vi "Sniffer.vi"() -> ()   [LabVIEW 2017]
uses:
  <vilib>/Instr/_visa.llb/VISA Open Access Mode.ctl
  <vilib>/Instr/_visa.llb/VISA Configure Serial Port (Instr).vi
panel:
  in  "Start":bool caption="Play Button"
  in  "Refresh Button":bool
  out "String":string
  in  "Stop Button":bool
  in  "flow control (0:none)":u16(ring) items=["None", "XON/XOFF", "RTS/CTS", "XON/XOFF & RTS/CTS", "DTR/DSR", "XON/XOFF & DTR/DSR"]
  in  "stop bits (10: 1 bit)":u16=10
  in  "parity (0:none)":u16(ring) items=["None", "Odd", "Even", "Mark", "Space"]
  in  "data bits (8)":u16=8 min=5 max=8 step=1
  in  "baud rate (9600)":u32=460800
  in  "Enable Termination\nChar (T)":bool
  in  "termination char\n(0xA = '\\n' = LF)":u8=10 format="%.0x"
  in  "timeout (10sec)":u32=100
  in  "VISA resource name":refnum<visa-resource-name>="COM3"
  # "V 0.1c"
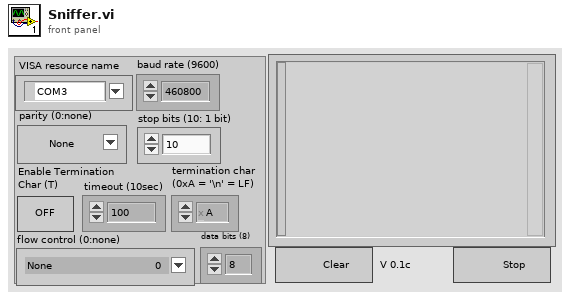
[diagram p1: front panel]
types:
  T1 = typedef "VISA Open Access Mode.ctl" = u32
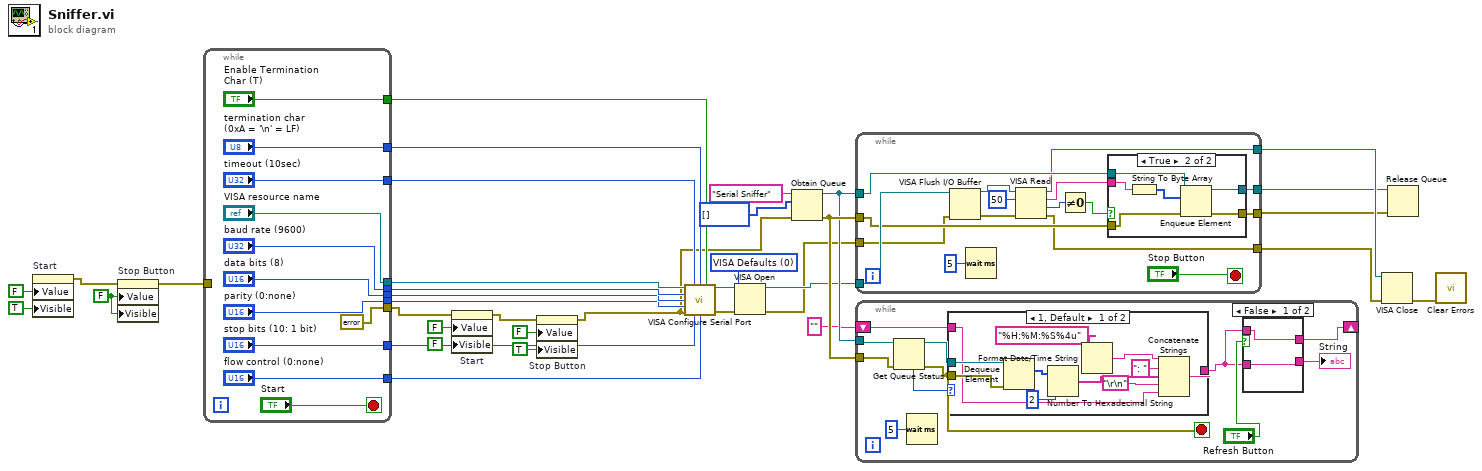
[diagram p0: block diagram]
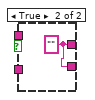
[diagram p2: hidden frame]
diagram:
  w12 = FALSE ("Stop Button")
  w25 = T1 0 items=["VISA Defaults"=0, "Exclusive Lock"=1, "Load Configured Settings"=4] ("Access Mode")
  n1 = property on="Start" class="Bool (strict)"("Value"=FALSE ("Start"), "Visible"=TRUE) -> (error out=w8:errorcluster)  [unwired: 2 in, 1 out]
  n2 = property on="Stop Button" class="Bool (strict)"(error in=w8, "Value"=w12, "Visible"=w12) -> (error out=w11:errorcluster)  [unwired: 1 in, 1 out]
  n3 = while {
    tunnel: ["VISA resource name"] -> w36
    tunnel: ["timeout (10sec)"] -> w35
    tunnel: ["termination char\n(0xA = '\\n' = LF)"] -> w34
    tunnel: ["baud rate (9600)"] -> w33
    tunnel: ["data bits (8)"] -> w32
    tunnel: ["parity (0:none)"] -> w31
    tunnel: ["stop bits (10: 1 bit)"] -> w30
    tunnel: ["flow control (0:none)"] -> w29
    tunnel: ["Enable Termination\nChar (T)"] -> w28
    tunnel: [errorcluster {"status"=FALSE, "code"=0, "source"=""} ("error in (no error)")] -> w3
    tunnel: w11 -> [_]
    stop <- "Start" stop-if-true
  }
  n4 = property on="Start" class="Bool (strict)"(error in=w3, "Value"=FALSE ("Start"), "Visible"=FALSE) -> (error out=w7:errorcluster)  [unwired: 1 in, 1 out]
  n5 = property on="Stop Button" class="Bool (strict)"(error in=w7, "Value"=FALSE ("Stop Button"), "Visible"=TRUE) -> (error out=w2:errorcluster)  [unwired: 1 in, 1 out]
  n6 = call-poly "VISA Configure Serial Port"("VISA resource name"=w36, "timeout (10sec)"=w35, "termination char\n(0xA = '\\n' = LF)"=w34, "Enable Termination\nChar (T)"=w28, "baud rate (9600)"=w33, "data bits (8)"=w32, "parity (0:none)"=w31, "error in (no error)"=w2, "stop bits (10: 1 bit)"=w30, "flow control (0:none)"=w29) -> ("VISA resource name out"=w27:refnum<visa-resource-name>, "error out"=w26:errorcluster)  [unwired: 4 in]
  n7 = VISA Open(access mode=w25, error in (no error)=w26, VISA resource name=w27) -> (VISA resource name=w21:refnum<visa-resource-name>, error out=w20:errorcluster)  [unwired: 2 in]
  n8 = Obtain Queue(name (unnamed)="Serial Sniffer", element data type=u8[] [], error in (no error)=w2) -> (queue out=w22:refnum<queue>, error out=w23:errorcluster)  [unwired: 2 in, 1 out]
  n9 = while {
    tunnel: w22 -> [w56]
    tunnel: w23 -> [w55]
    tunnel: w21 -> [w61]
    tunnel: [w54] -> w17
    tunnel: w20 -> [w53]
    tunnel: [w51] -> w19
    tunnel: [w50] -> w18
    tunnel: [w49] -> w16
    stop <- "Stop Button" stop-if-true
    n10 = VISA Flush I/O Buffer(VISA resource name=w61, error in (no error)=w53) -> (VISA resource name out=w62:refnum<visa-resource-name>, error out=w60:errorcluster)  [unwired: 1 in]
    n11 = Wait (ms)(milliseconds to wait=u32 5) -> ()  [unwired: 1 out]
    n12 = VISA Read(VISA resource name=w62, byte count=u32 50, error in (no error)=w60) -> (VISA resource name out=w50:refnum<visa-resource-name>, read buffer=w57:string, return count=w59:u32, error out=w51:errorcluster)
    n13 = Not Equal To 0?(x=w59) -> (x != 0?=w58:bool)
    n14 = case shown="True" w58 {
      tunnel: w57 -> [_ w67]
      tunnel: w56 -> [w64 w71]
      tunnel: w55 -> [w65 w70]
      tunnel: [w65 w69] -> w54
      tunnel: [w64 w68] -> w49
      frame False {
      }
      frame True {
        n15 = String To Byte Array(string=w67) -> (unsigned byte array=w66:u8[])
        n16 = Enqueue Element(queue=w71, element=w66, error in (no error)=w70) -> (queue out=w68:refnum<queue>, error out=w69:errorcluster)  [unwired: 1 in, 1 out]
      }
    }
  }
  n17 = while {
    tunnel: w23 -> [w81]
    tunnel: w22 -> [w82]
    shift-right: [w74] -> _
    shift-left: "" -> [w78]
    stop <- w77 stop-if-true
    n18 = Get Queue Status(queue=w82, error in (no error)=w81) -> (queue out=w79:refnum<queue>, error out=w77:errorcluster, # elements in queue=w80:i32)  [unwired: 1 in, 5 out]
    n19 = Wait (ms)(milliseconds to wait=u32 5) -> ()  [unwired: 1 out]
    n20 = case shown="1, Default" w80 {
      tunnel: w79 -> [w96 _]
      tunnel: w77 -> [w95 _]
      tunnel: [w94 w97] -> w73
      tunnel: w78 -> [w89 w97]
      frame 1, Default {
        n21 = Dequeue Element(queue=w96, error in (no error)=w95) -> (element=w92:u8[])  [unwired: 1 in, 3 out]
        n22 = Number To Hexadecimal String(1:i16 2 ("width (-)"), 2:w92) -> (0:w91:string[])
        n23 = Format Date/Time String(time format string (%c)="%H:%M:%S%4u") -> (date/time string=w86:string)  [unwired: 2 in]
        n24 = Concatenate Strings(w86, ": " ("string"), w91, "\r\n", w89) -> (w94:string)
      }
      frame 0 {
      }
    }
    n25 = case shown="False" "Refresh Button" {
      tunnel: w73 -> [w83 _]
      tunnel: [w83 w85] -> w75
      tunnel: [w84 w85] -> w74
      tunnel: w73 -> [w84 _]
      frame False {
      }
      frame True {
        w85 = ""
      }
    }
    "String" <- w75
  }
  n26 = VISA Close(VISA resource name=w18, error in (no error)=w19) -> (error out=w14:errorcluster)
  n27 = Release Queue(queue=w16, error in (no error)=w17) -> ()  [unwired: 1 in, 3 out]
  n28 = call <vilib>:"Clear Errors.vi"("error in (no error)"=w14) -> ()  [unwired: 5 in, 2 out]
